vi "SMR_LabVIEW_V4.5.vi"() -> ()   [LabVIEW 2025]
uses:
  <vilib>/DAQmx/write.llb/DAQmx Write (Analog DBL 1Chan 1Samp).vi
  <vilib>/DAQmx/read.llb/DAQmx Read (Analog 1D DBL NChan 1Samp).vi
  <vilib>/DAQmx/create/channels.llb/DAQmx Create Channel (AI-Temperature-Thermocouple).vi
  <vilib>/DAQmx/create/channels.llb/DAQmx Create Channel (AI-Voltage-Basic).vi
  <vilib>/DAQmx/create/channels.llb/DAQmx Create Channel (AO-Voltage-Basic).vi
  <vilib>/DAQmx/miscellaneous.llb/DAQmx Fill In Error Info.vi
panel:
  out "Valve Output Voltage (V)":dbl
  out "Valve Command Final (%)":dbl
  in  "Valve Output Enable":bool
  in  "Manual Valve Control (%)":dbl min=0.0 max=100.0
  out "Heat Exchanger Pressure History":dbl(graph)
  out "Main Loop Pressure History":T1(graph)
  out "Heat Exchanger Temperature History":cluster{"Waveform":dbl, "Waveform":dbl}(graph)
  out "Main Loop Temeperature History":T2(graph)
  out "Overall Avg Pressure (psi)":dbl
  out "Heat Exchanger Pressure P6 (psi)":dbl
  out "Main Loop Avg Pressure (psi)":dbl
  out "Heat Exchanger Avg Temp (deg C)":dbl
  out "Main Loop Avg Temp (deg C)":dbl
  out "Raw NI9201 \nVoltage Display":T3
  out "Temperature Display":T4
  out "Pressure Display":T5
  in  "Flow Offset Correction (GPM)":dbl=-0.3
  out "Flow History":dbl(graph)
  out "Overall Pressure History":T6(graph)
  out "Overall Temperature History":T7(graph)
  out "Max Loop Pressure (psi)":dbl
  out "Overall Avg Temp (deg C)":dbl
  out "Max Loop Temp (deg C)":dbl
  out "Heat Exchanger Flow (GPM)":dbl
  in  "Loop Period (ms)":dbl=1000.0
  in  "Stop":bool
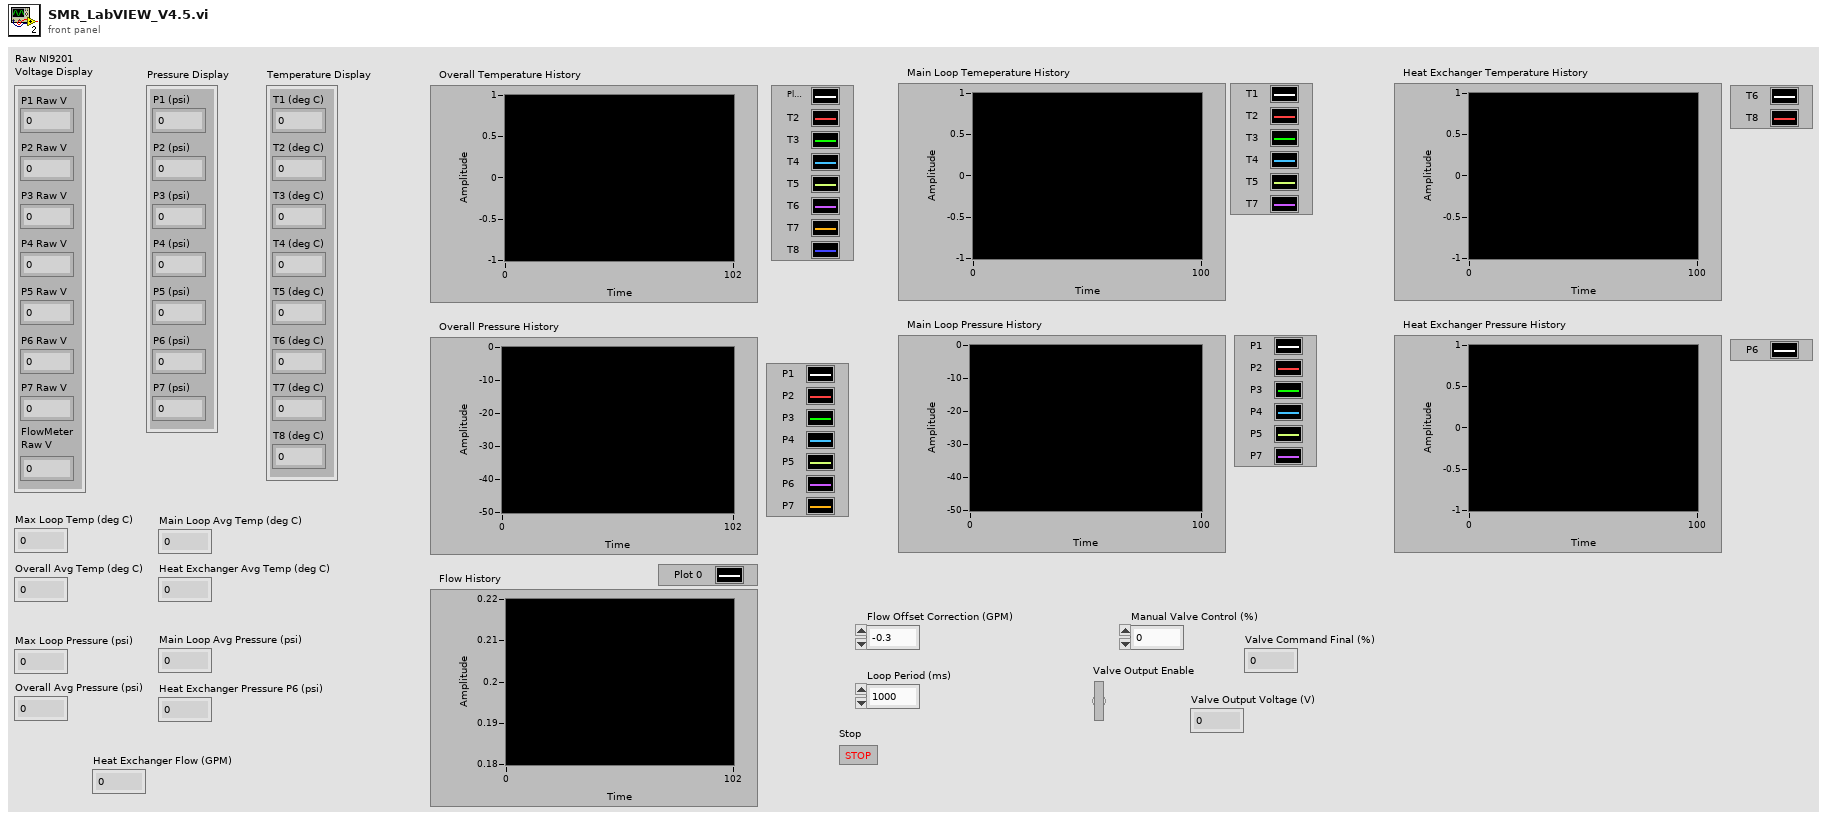
[diagram p1: front panel]
types:
  T1 = cluster{"P1":dbl, "P2":dbl, "P3":dbl, "P4":dbl, "P5":dbl, "P7":dbl}
  T2 = cluster{"Waveform":dbl, "Waveform":dbl, "Waveform":dbl, "Waveform":dbl, "Waveform":dbl, "Waveform":dbl}
  T3 = cluster{"P1 Raw V":dbl, "P2 Raw V":dbl, "P3 Raw V":dbl, "P4 Raw V":dbl, "P5 Raw V":dbl, "P6 Raw V":dbl, "P7 Raw V":dbl, "FlowMeter\nRaw V":dbl}
  T4 = cluster{"T1 (deg C)":dbl, "T2 (deg C)":dbl, "T3 (deg C)":dbl, "T4 (deg C)":dbl, "T5 (deg C)":dbl, "T6 (deg C)":dbl, "T7 (deg C)":dbl, "T8 (deg C)":dbl}
  T5 = cluster{"P1 (psi)":dbl, "P2 (psi)":dbl, "P3 (psi)":dbl, "P4 (psi)":dbl, "P5 (psi)":dbl, "P6 (psi)":dbl, "P7 (psi)":dbl}
  T6 = cluster{"P1":dbl, "P2":dbl, "P3":dbl, "P4":dbl, "P5":dbl, "P6":dbl, "P7":dbl}
  T7 = cluster{"Waveform":dbl, "Waveform":dbl, "Waveform":dbl, "Waveform":dbl, "Waveform":dbl, "Waveform":dbl, "Waveform":dbl, "Waveform":dbl}
  T8 = cluster{"P1":dbl, "P2":dbl, "P3":dbl, "P4":dbl, "P5":dbl, "P6":dbl, "P7":dbl, "Flow":dbl}
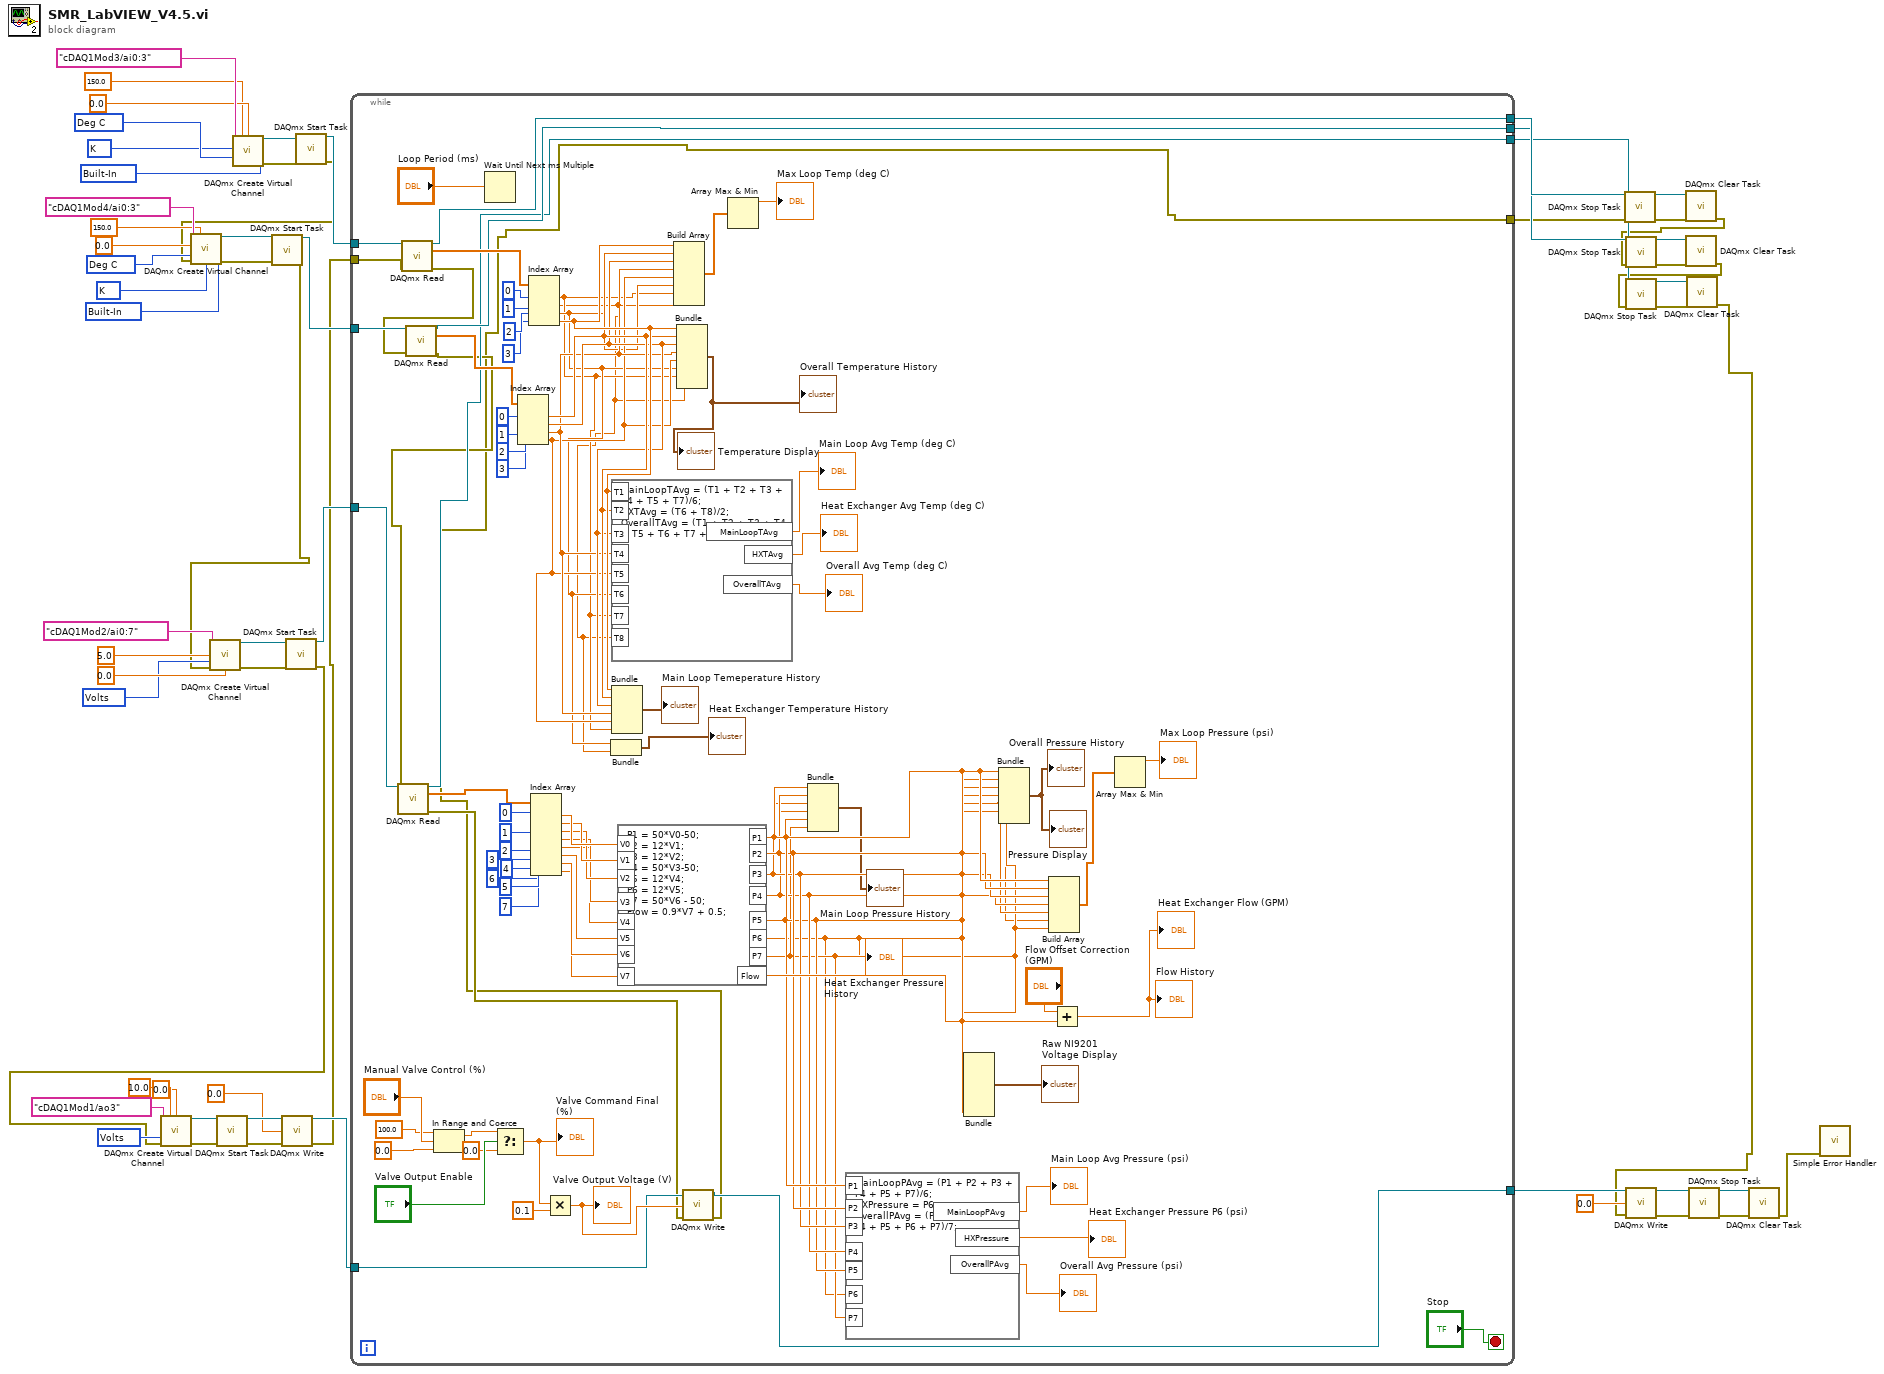
[diagram p0: block diagram]
diagram:
  w19 = 10348 items=["Volts"=10348, "From Custom Scale"=10065] ("units")
  w41 = 10348 items=["Volts"=10348, "From Custom Scale"=10065] ("units")
  w45 = 10200 items=["Built-In"=10200, "Constant Value"=10116, "Channel"=10113] ("cjc source")
  w46 = 10073 items=["J"=10072, "K"=10073, "N"=10077, "R"=10082, "S"=10085, "T"=10086, "B"=10047, "E"=10055] ("thermocouple type")
  w29 = 10143 items=["Deg C"=10143, "Deg F"=10144, "Kelvins"=10325, "Deg R"=10145, "From Custom Scale"=10065] ("units")
  w49 = 10200 items=["Built-In"=10200, "Constant Value"=10116, "Channel"=10113] ("cjc source")
  w50 = 10073 items=["J"=10072, "K"=10073, "N"=10077, "R"=10082, "S"=10085, "T"=10086, "B"=10047, "E"=10055] ("thermocouple type")
  w53 = 10143 items=["Deg C"=10143, "Deg F"=10144, "Kelvins"=10325, "Deg R"=10145, "From Custom Scale"=10065] ("units")
  n1 = call-poly <vilib>:"DAQmx Create Virtual Channel.vi"("maximum value"=150.0, "minimum value"=0.0, "physical channels"=tag "cDAQ1Mod3/ai0:3", "cjc source"=w49, "units"=w53, "thermocouple type"=w50) -> ("task out"=w58:refnum<k21>, "error out"=w57:errorcluster)  [unwired: 8 in]
  n2 = call <vilib>:"DAQmx Start Task.vi"("task/channels in"=w58, "error in"=w57) -> ("task out"=w38:refnum<k21>, "error out"=w28:errorcluster)  [unwired: 12 in]
  n3 = call-poly <vilib>:"DAQmx Create Virtual Channel.vi"("maximum value"=150.0, "minimum value"=0.0, "physical channels"=tag "cDAQ1Mod4/ai0:3", "cjc source"=w45, "units"=w29, "error in"=w28, "thermocouple type"=w46) -> ("task out"=w55:refnum<k21>, "error out"=w54:errorcluster)  [unwired: 7 in]
  n4 = call <vilib>:"DAQmx Start Task.vi"("task/channels in"=w55, "error in"=w54) -> ("task out"=w37:refnum<k21>, "error out"=w27:errorcluster)  [unwired: 12 in]
  n5 = call-poly <vilib>:"DAQmx Create Virtual Channel.vi"("maximum value"=5.0, "minimum value"=0.0, "physical channels"=tag "cDAQ1Mod2/ai0:7", "units"=w41, "error in"=w27) -> ("task out"=w40:refnum<k21>, "error out"=w39:errorcluster)  [unwired: 9 in]
  n6 = call <vilib>:"DAQmx Start Task.vi"("task/channels in"=w40, "error in"=w39) -> ("task out"=w36:refnum<k21>, "error out"=w6:errorcluster)  [unwired: 12 in]
  n7 = call-poly <vilib>:"DAQmx Create Virtual Channel.vi"("maximum value"=10.0, "minimum value"=0.0, "physical channels"=tag "cDAQ1Mod1/ao3", "units"=w19, "error in"=w6) -> ("task out"=w18:refnum<k21>, "error out"=w17:errorcluster)  [unwired: 9 in]
  n8 = call <vilib>:"DAQmx Start Task.vi"("task/channels in"=w18, "error in"=w17) -> ("task out"=w16:refnum<k21>, "error out"=w15:errorcluster)  [unwired: 12 in]
  n9 = call-poly <vilib>:"DAQmx Write.vi"("task/channels in"=w16, "data"=0.0, "error in"=w15) -> ("task out"=w13:refnum<k21>, "error out"=w5:errorcluster)  [unwired: 10 in, 1 out]
  n10 = while {
    tunnel: w38 -> [w142]
    tunnel: w37 -> [w141]
    tunnel: w36 -> [w128]
    tunnel: [w109] -> w35
    tunnel: [w108] -> w34
    tunnel: [w107] -> w33
    tunnel: w5 -> [w106]
    tunnel: [w60] -> w26
    tunnel: w13 -> [w63]
    tunnel: [w62] -> w12
    stop <- "Stop" stop-if-true
    n11 = call-poly <vilib>:"DAQmx Read.vi"("task/channels in"=w142, "error in"=w106) -> ("task out"=w109:refnum<k21>, "data"=w132:dbl[], "error out"=w105:errorcluster)  [unwired: 11 in]
    n12 = call-poly <vilib>:"DAQmx Read.vi"("task/channels in"=w141, "error in"=w105) -> ("task out"=w108:refnum<k21>, "data"=w131:dbl[], "error out"=w104:errorcluster)  [unwired: 11 in]
    n13 = call-poly <vilib>:"DAQmx Read.vi"("task/channels in"=w128, "error in"=w104) -> ("task out"=w107:refnum<k21>, "data"=w119:dbl[], "error out"=w61:errorcluster)  [unwired: 11 in]
    n14 = In Range and Coerce(upper limit=100.0, x="Manual Valve Control (%)", lower limit=0.0) -> (coerced(x)=w68:dbl)  [unwired: 1 out]
    n15 = Wait Until Next ms Multiple(millisecond multiple="Loop Period (ms)") -> ()  [unwired: 1 out]
    n16 = Select(t=w68, s="Valve Output Enable", f=0.0) -> (s? t:f=w65:dbl)
    "Valve Command Final (%)" <- w65
    n17 = Index Array(array=w131, index #1=0 ("index"), index #2=1 ("index"), index #3=2 ("index"), index #4=3 ("index")) -> (element #1=w89:dbl, element #2=w88:dbl, element #3=w87:dbl, element #4=w86:dbl)
    n18 = Index Array(array=w132, index #1=0 ("index"), index #2=1 ("index"), index #3=2 ("index"), index #4=3 ("index")) -> (element #1=w83:dbl, element #2=w82:dbl, element #3=w84:dbl, element #4=w90:dbl)
    n19 = Index Array(array=w119, index #1=0 ("index"), index #2=1 ("index"), index #3=2 ("index"), index #4=3 ("index"), index #5=4 ("index"), index #6=5 ("index"), index #7=6 ("index"), index #8=7 ("index")) -> (element #1=w118:dbl, element #2=w117:dbl, element #3=w116:dbl, element #4=w115:dbl, element #5=w114:dbl, element #6=w113:dbl, element #7=w112:dbl, element #8=w111:dbl)
    n20 = Multiply(x=w65, y=0.1) -> (x*y=w64:dbl)
    "Valve Output Voltage (V)" <- w64
    n21 = Bundle("Waveform"=w84, "Waveform"=w82) -> (→"Heat Exchanger Temperature History":cluster{"Waveform":dbl, "Waveform":dbl})  [unwired: 1 in]
    n22 = formula code="MainLoopTAvg = (T1 + T2 + T3 + T4 + T5 + T7)/6;\nHXTAvg = (T6 + T8)/2;\nOverallTAvg = (T1 + T2 + T3 + T4 + T5 + T6 + T7 + T8)/8;"("T1"=w90, "T2"=w89, "T3"=w88, "T4"=w87, "T5"=w86, "T6"=w84, "T7"=w83, "T8"=w82) -> ("MainLoopTAvg"=→"Main Loop Avg Temp (deg C)":dbl, "HXTAvg"=→"Heat Exchanger Avg Temp (deg C)":dbl, "OverallTAvg"=→"Overall Avg Temp (deg C)":dbl)
    n23 = Bundle("Waveform"=w90, "Waveform"=w89, "Waveform"=w88, "Waveform"=w87, "Waveform"=w86, "Waveform"=w83) -> (→"Main Loop Temeperature History":T2)  [unwired: 1 in]
    n24 = formula code="P1 = 50*V0-50;\nP2 = 12*V1;\nP3 = 12*V2;\nP4 = 50*V3-50;\nP5 = 12*V4;\nP6 = 12*V5; \nP7 = 50*V6 - 50;\nFlow = 0.9*V7 + 0.5;"("V0"=w118, "V1"=w117, "V2"=w116, "V3"=w115, "V4"=w114, "V5"=w113, "V6"=w112, "V7"=w111) -> ("P1"=w80:dbl, "P2"=w79:dbl, "P3"=w78:dbl, "P4"=w77:dbl, "P5"=w76:dbl, "P6"=w73:dbl, "P7"=w75:dbl, "Flow"=w98:dbl)
    "Heat Exchanger Pressure History" <- w73
    n25 = Build Array(w90, w89, w88, w87, w86, w84, w83, w82) -> (w129:dbl[])
    n26 = Bundle("Waveform"=w90, "Waveform"=w89, "Waveform"=w88, "Waveform"=w87, "Waveform"=w86, "Waveform"=w84, "Waveform"=w83, "Waveform"=w82) -> (→"Overall Temperature History" →"Temperature Display":T7)  [unwired: 1 in]
    n27 = call-poly <vilib>:"DAQmx Write.vi"("task/channels in"=w63, "data"=w64, "error in"=w61) -> ("task out"=w62:refnum<k21>, "error out"=w60:errorcluster)  [unwired: 10 in, 1 out]
    n28 = Array Max & Min(array=w129) -> (max value=→"Max Loop Temp (deg C)":dbl)  [unwired: 3 out]
    n29 = Bundle("P1"=w80, "P2"=w79, "P3"=w78, "P4"=w77, "P5"=w76, "P7"=w75) -> (→"Main Loop Pressure History":T1)  [unwired: 1 in]
    n30 = formula code="MainLoopPAvg = (P1 + P2 + P3 + P4 + P5 + P7)/6;\nHXPressure = P6;\nOverallPAvg = (P1 + P2 + P3 + P4 + P5 + P6 + P7)/7;"("P1"=w80, "P2"=w79, "P3"=w78, "P4"=w77, "P5"=w76, "P6"=w73, "P7"=w75) -> ("MainLoopPAvg"=→"Main Loop Avg Pressure (psi)":dbl, "HXPressure"=→"Heat Exchanger Pressure P6 (psi)":dbl, "OverallPAvg"=→"Overall Avg Pressure (psi)":dbl)
    n31 = Bundle("P1"=w80, "P2"=w79, "P3"=w78, "P4"=w77, "P5"=w76, "P6"=w73, "P7"=w75, "Flow"=w98) -> (→"Raw NI9201 \nVoltage Display":T8)  [unwired: 1 in]
    n32 = Bundle("P1"=w80, "P2"=w79, "P3"=w78, "P4"=w77, "P5"=w76, "P6"=w73, "P7"=w75) -> (→"Overall Pressure History" →"Pressure Display":T6)  [unwired: 1 in]
    n33 = Build Array(w80, w79, w78, w77, w76, w73, w75) -> (w101:dbl[])
    n34 = Add(x="Flow Offset Correction (GPM)", y=w98) -> (x+y=→"Heat Exchanger Flow (GPM)" →"Flow History":dbl)
    n35 = Array Max & Min(array=w101) -> (max value=→"Max Loop Pressure (psi)":dbl)  [unwired: 3 out]
  }
  n36 = call <vilib>:"DAQmx Stop Task.vi"("task/channels in"=w35, "error in"=w26) -> ("task out"=w32:refnum<k21>, "error out"=w25:errorcluster)  [unwired: 12 in]
  n37 = call <vilib>:"DAQmx Clear Task.vi"("task in"=w32, "error in"=w25) -> ("error out"=w4:errorcluster)  [unwired: 13 in]
  n38 = call <vilib>:"DAQmx Stop Task.vi"("task/channels in"=w34, "error in"=w4) -> ("task out"=w31:refnum<k21>, "error out"=w24:errorcluster)  [unwired: 12 in]
  n39 = call <vilib>:"DAQmx Clear Task.vi"("task in"=w31, "error in"=w24) -> ("error out"=w3:errorcluster)  [unwired: 13 in]
  n40 = call <vilib>:"DAQmx Stop Task.vi"("task/channels in"=w33, "error in"=w3) -> ("task out"=w30:refnum<k21>, "error out"=w23:errorcluster)  [unwired: 12 in]
  n41 = call <vilib>:"DAQmx Clear Task.vi"("task in"=w30, "error in"=w23) -> ("error out"=w2:errorcluster)  [unwired: 13 in]
  n42 = call-poly <vilib>:"DAQmx Write.vi"("task/channels in"=w12, "data"=0.0, "error in"=w2) -> ("task out"=w10:refnum<k21>, "error out"=w9:errorcluster)  [unwired: 10 in, 1 out]
  n43 = call <vilib>:"DAQmx Stop Task.vi"("task/channels in"=w10, "error in"=w9) -> ("task out"=w8:refnum<k21>, "error out"=w7:errorcluster)  [unwired: 12 in]
  n44 = call <vilib>:"DAQmx Clear Task.vi"("task in"=w8, "error in"=w7) -> ("error out"=w1:errorcluster)  [unwired: 13 in]
  n45 = call <vilib>:"Simple Error Handler.vi"("error in (no error)"=w1) -> ()  [unwired: 4 in, 5 out]
